vi "init.vi"(8 "error in (no error)":errorcluster, 10 "Config":string, 11 "Serial in":refnum<class "Serial.lvclass">) -> (0 "error out":errorcluster, 3 "Serial out":refnum<class "Serial.lvclass">)   [LabVIEW 2015, in "Serializer.lvlib" / "Serial.lvclass"]
uses:
  Serial.lvclass
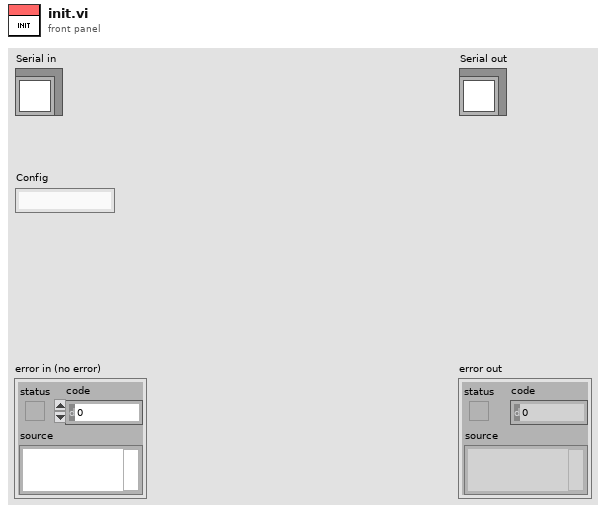
[diagram p1: front panel]
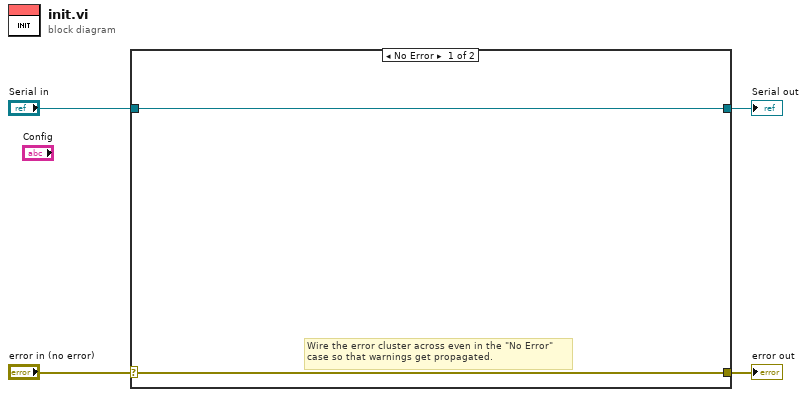
[diagram p0: block diagram]
diagram:
  n1 = case shown="No Error" "error in (no error)" {
    selector: "error in (no error)" -> [w5 w8]
    tunnel: [w5 w8] -> w3
    tunnel: [w6 w7] -> w1
    tunnel: "Serial in" -> [w6 w7]
    frame No Error {
      # "Wire the error cluster across even in the \"No Error\"\ncase so that warnings get propagated."
    }
    frame Error {
    }
  }
  "error out" <- w3
  "Serial out" <- w1
